vi "Red's Auto Clicker.vi"(8 "error in (no error)":errorcluster) -> (0 "error out":errorcluster)   [LabVIEW 2023]
doc: "Presents an interface to create, edit, save, and execute user-defined macros."
uses:
  CTLs/State Data.ctl
  CTLs/Macro Cluster V3.ctl
  CTLs/Macro Config V3.ctl
  CTLs/Step V3.ctl
  CTLs/Step Type V3.ctl
  CTLs/Hotkey Values.ctl
  CTLs/Refs.ctl
  <vilib>/Utility/miscctls.llb/LVRowAndColumnUnsignedTypeDef.ctl
  CTLs/FGV Actions.ctl
  CTLs/Hotkey Type.ctl
  bd503c13-d10c-440e-ab5e-4e60baef5deb.vi
  <vilib>/Utility/inputDevices.llb/closeKeyboard.vi
  SubVIs/FaKI State Machine/FaKI State Machine.lvlib
panel:
  out "Status":string
  in  "Add Step 2":bool
  in  "Dbl Click":T1
  in  "Macro Steps":i32(listbox)
  out "Abort Hotkey":string caption="Abort Hotkey:"
  out "Metadata":string
  in  "Description":string
  out "Resolutions":cluster{"Width":i16, "Height":i16}[](array[cluster])
  out "n Monitors":i32
  in  "Settings":bool
  in  "Export":bool
  in  "Import":bool
  out "Macro Hotkey":string caption="Macro Hotkey:"
  in  "Delete":bool
  in  "Start/Stop":bool
  in  "N":i32 caption="Times to Repeat\n(-1 = indefinitely)" min=-1
  in  "Activation Type":enum32{"Hotkey", "Automatic"}(radio)
  out "Row":i32
  in  "Clear Steps":bool
  in  "Delete Step":bool
  in  "Insert Step":bool
  in  "Add Step":bool
  in  "Modify Step":bool
  in  "Exit":bool
  in  "Save":bool
  in  "Restore":bool
  in  "Help":bool
  in  "Macro Name":string(combo)
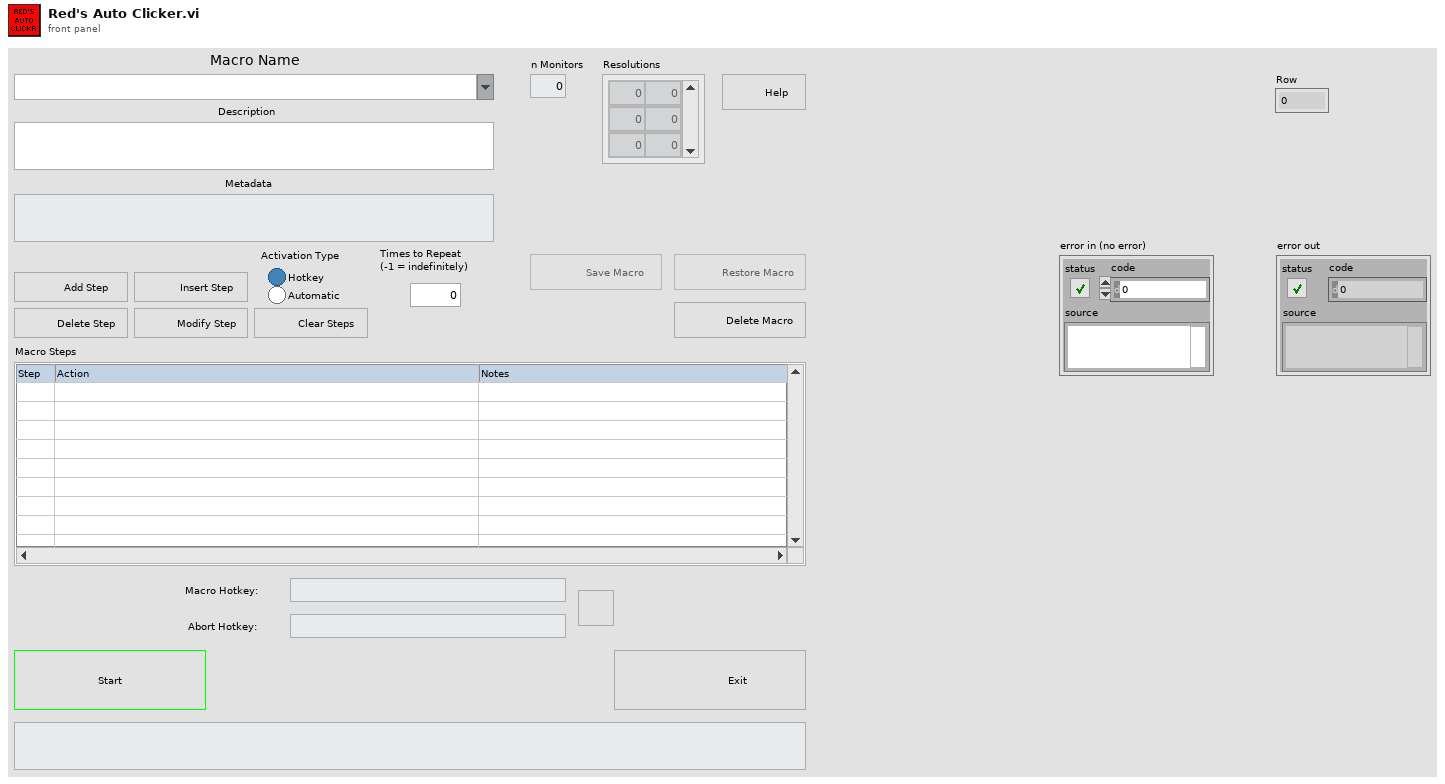
[diagram p1: front panel]
types:
  T1 = cluster{"Insert Before":bool, "Insert After":bool, "Modify Step 2":bool, "Delete Step 2":bool}
  T2 = typedef "LVPoint32TypeDef.ctl" = cluster{"Horizontal":i32, "Vertical":i32}
  T3 = enum32{"Invalid", "Standard", "Closed", "Hidden", "Minimized", "Maximized"}
  T4 = enum32{"invalid app kind", "Development System", "Run Time System", "Student Edition", "Embedded LabVIEW", "Evaluation", "Custom"}
  T5 = typedef "State Data.ctl" = cluster{"Core":cluster{"Current VI Reference":refnum<vi>, "Close Panel on Exit?":bool}, "Macro":cluster{"New":T6, "Saved":T6, "Name":string}, "Step":i32, "n":i32, "Hotkey Values":T10, "Keyboard":refnum<k1>, "Macro Active?":bool, "Macro Names":string[], "Rcount":i32, "Refs":T11, "Resolutions":cluster{"Width":i16, "Height":i16}[], "App Data Dir":path, "Start Time":timestamp}
  T6 = typedef "Macro Cluster V3.ctl" = cluster{"Config":T7, "Steps":T8[]}
  T7 = typedef "Macro Config V3.ctl" = cluster{"Schema Version":string, "Activation Type":enum32{"Hotkey", "Automatic"}, "N":i32, "Description":string, "Resolutions":cluster{"Width":i16, "Height":i16}[], "Date Created":timestamp, "Date Updated":timestamp}
  T8 = typedef "Step V3.ctl" = cluster{"Type":T9, "X":i32, "Y":i32, "Delay":i32, "Key":u8, "Repeat":i32, "RClick?":bool, "App/Window Name":string, "Notes":string}
  T9 = typedef "Step Type V3.ctl" = enum16{"Mouse Move", "Mouse Click", "Key Press", "Wait", "Mouse Down", "Mouse Up", "Key Down", "Key Up", "Run Application", "Maximize Window", "Restore Window", "Minimize Window", "Close Window", "Bring Window to Front", "Send Window to Back"}
  T10 = typedef "Hotkey Values.ctl" = cluster{"Macro Hotkey":enum16{"0", "1", "2", "3", "4", "5", "6", "7", "8", "9", "A", "B", "C", "D", "E", "F", "G", "H", "I", "J", "K", "L", "M", "N", "O", "P", "Q", "R", "S", "T", "U", "V", "W", "X", "Y", "Z", "F1", "F2", "F3", "F4", "F5", "F6", "F7", "F8", "F9", "F10", "F11", "F12", "F13", "F14", "F15", "ADD", "BACK", "BACKSLASH", "CAPITAL", "COMMA", "DECIMAL", "DELETE", "DIVIDE", "DOWN", "END", "EQUALS", "ESCAPE", "GRAVE (`)", "HOME", "INSERT", "LBRACKET", "LCONTROL", "LEFT", "L ALT", "LSHIFT", "LWIN", "MINUS", "MULTIPLY", "NEXT", "NUMLOCK", "NUMPAD_0", "NUMPAD_1", "NUMPAD_2", "NUMPAD_3", "NUMPAD_4", "NUMPAD_5", "NUMPAD_6", "NUMPAD_7", "NUMPAD_8", "NUMPAD_9", "PAUSE", "PERIOD", "PRIOR (PG UP)", "RBRACKET", "RCONTROL", "RETURN", "RIGHT", "R ALT", "RSHIFT", "RWIN", "SCROLL", "SEMICOLON", "SLASH", "SPACE", "SUBTRACT", "TAB", "UP", "ENTER (num pad)", "' (quote)"}[], "Abort Hotkey":enum16{"0", "1", "2", "3", "4", "5", "6", "7", "8", "9", "A", "B", "C", "D", "E", "F", "G", "H", "I", "J", "K", "L", "M", "N", "O", "P", "Q", "R", "S", "T", "U", "V", "W", "X", "Y", "Z", "F1", "F2", "F3", "F4", "F5", "F6", "F7", "F8", "F9", "F10", "F11", "F12", "F13", "F14", "F15", "ADD", "BACK", "BACKSLASH", "CAPITAL", "COMMA", "DECIMAL", "DELETE", "DIVIDE", "DOWN", "END", "EQUALS", "ESCAPE", "GRAVE (`)", "HOME", "INSERT", "LBRACKET", "LCONTROL", "LEFT", "L ALT", "LSHIFT", "LWIN", "MINUS", "MULTIPLY", "NEXT", "NUMLOCK", "NUMPAD_0", "NUMPAD_1", "NUMPAD_2", "NUMPAD_3", "NUMPAD_4", "NUMPAD_5", "NUMPAD_6", "NUMPAD_7", "NUMPAD_8", "NUMPAD_9", "PAUSE", "PERIOD", "PRIOR (PG UP)", "RBRACKET", "RCONTROL", "RETURN", "RIGHT", "R ALT", "RSHIFT", "RWIN", "SCROLL", "SEMICOLON", "SLASH", "SPACE", "SUBTRACT", "TAB", "UP", "ENTER (num pad)", "' (quote)"}[]}
  T11 = typedef "Refs.ctl" = cluster{"Name":refnum<vi>, "Description":refnum<vi>, "Import":refnum<vi>, "Export":refnum<vi>, "Delete":refnum<vi>, "Restore":refnum<vi>, "Save":refnum<vi>, "Start":refnum<vi>, "Steps":refnum<vi>, "Simple Refs":refnum<vi>[]}
  T12 = enum8{"Enabled", "Disabled", "Disabled and Grayed Out"}
  T13 = typedef "LVRowAndColumnUnsignedTypeDef.ctl" = cluster{"Row":u32, "Column":u32}
  T14 = typedef "Hotkey Type.ctl" = enum16{"Macro Hotkey", "Abort Hotkey"}
  T15 = typedef "FGV Actions.ctl" = enum16{"Read", "Write"}
  T16 = cluster{"Current VI Reference":refnum<vi>, "Close Panel on Exit?":bool}
  T17 = enum16{"0", "1", "2", "3", "4", "5", "6", "7", "8", "9", "A", "B", "C", "D", "E", "F", "G", "H", "I", "J", "K", "L", "M", "N", "O", "P", "Q", "R", "S", "T", "U", "V", "W", "X", "Y", "Z", "F1", "F2", "F3", "F4", "F5", "F6", "F7", "F8", "F9", "F10", "F11", "F12", "F13", "F14", "F15", "ADD", "BACK", "BACKSLASH", "CAPITAL", "COMMA", "DECIMAL", "DELETE", "DIVIDE", "DOWN", "END", "EQUALS", "ESCAPE", "GRAVE (`)", "HOME", "INSERT", "LBRACKET", "LCONTROL", "LEFT", "L ALT", "LSHIFT", "LWIN", "MINUS", "MULTIPLY", "NEXT", "NUMLOCK", "NUMPAD_0", "NUMPAD_1", "NUMPAD_2", "NUMPAD_3", "NUMPAD_4", "NUMPAD_5", "NUMPAD_6", "NUMPAD_7", "NUMPAD_8", "NUMPAD_9", "PAUSE", "PERIOD", "PRIOR (PG UP)", "RBRACKET", "RCONTROL", "RETURN", "RIGHT", "R ALT", "RSHIFT", "RWIN", "SCROLL", "SEMICOLON", "SLASH", "SPACE", "SUBTRACT", "TAB", "UP", "ENTER (num pad)", "' (quote)"}[]
  T18 = typedef "LVAllMonitorsDisplayTypeDef.ctl" = cluster{"Bounds":cluster{"Left":i16, "Top":i16, "Right":i16, "Bottom":i16}, "Depth":i16}[]
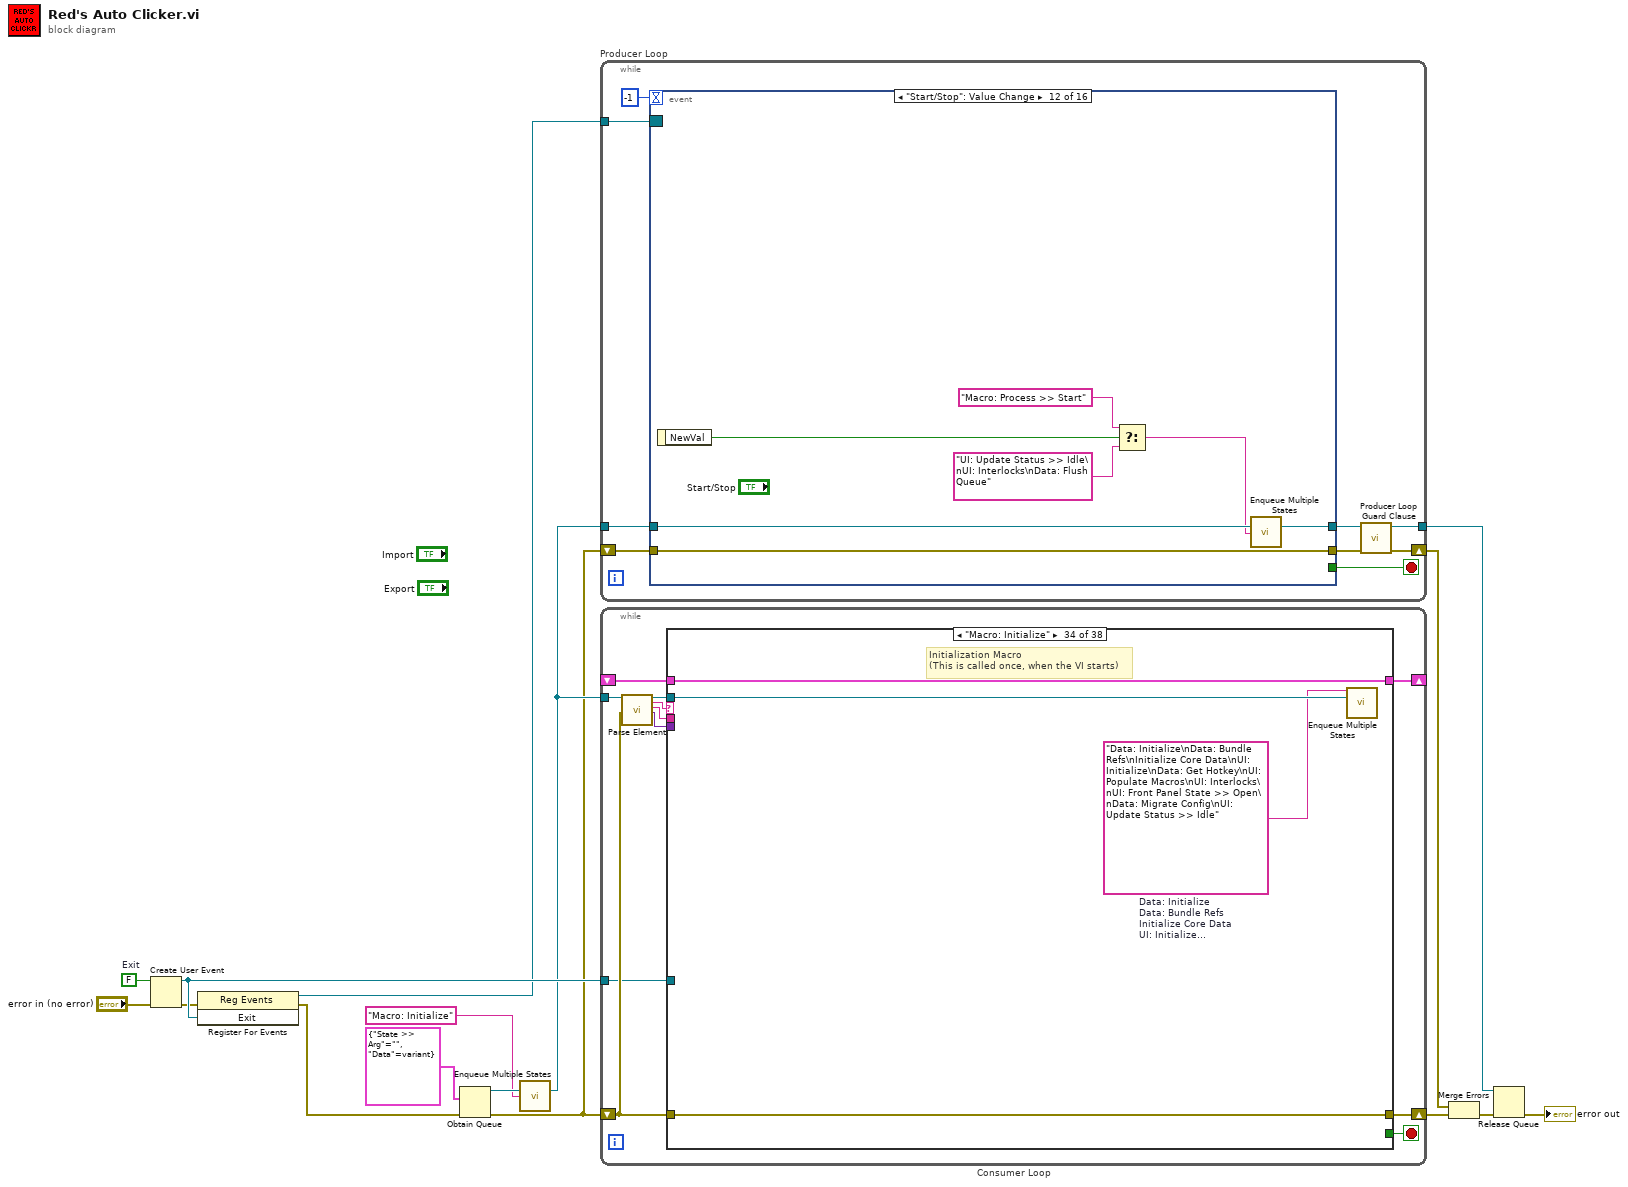
[diagram p0: block diagram]
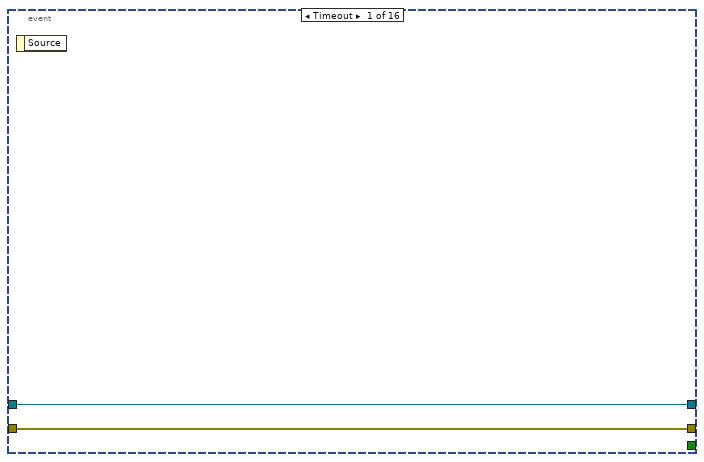
[diagram p2: hidden frame]
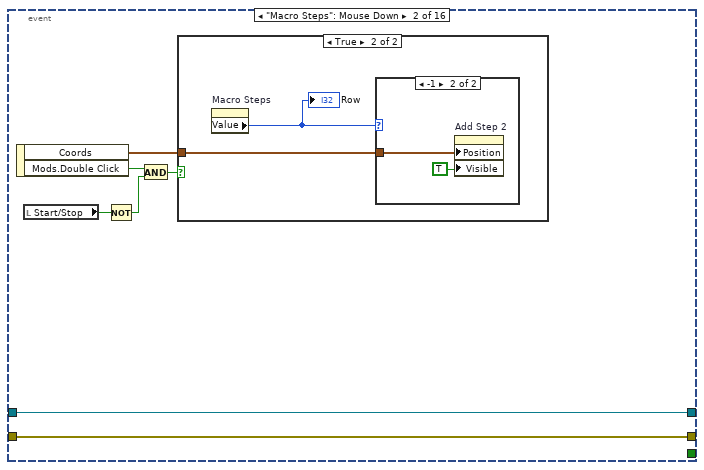
[diagram p3: hidden frame]
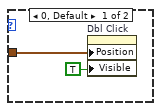
[diagram p5: hidden frame]
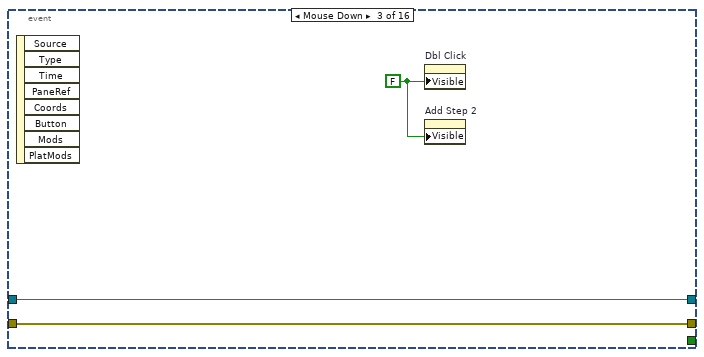
[diagram p6: hidden frame]
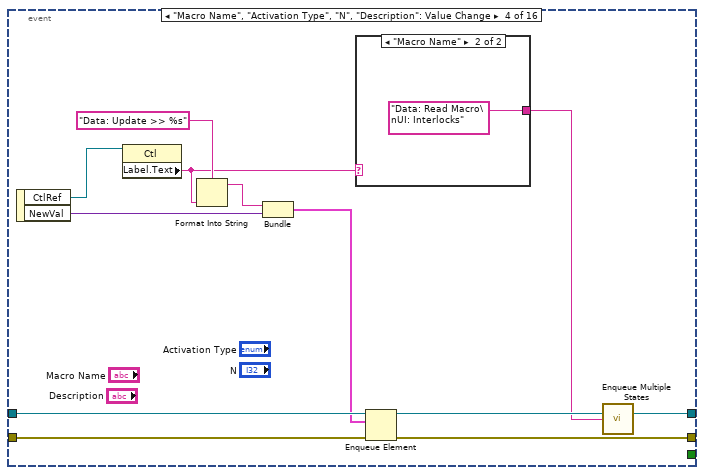
[diagram p7: hidden frame]
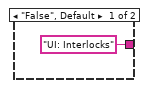
[diagram p8: hidden frame]
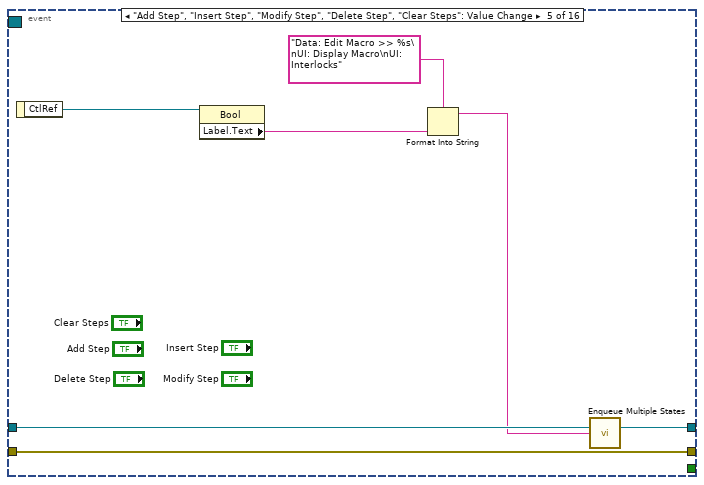
[diagram p9: hidden frame]
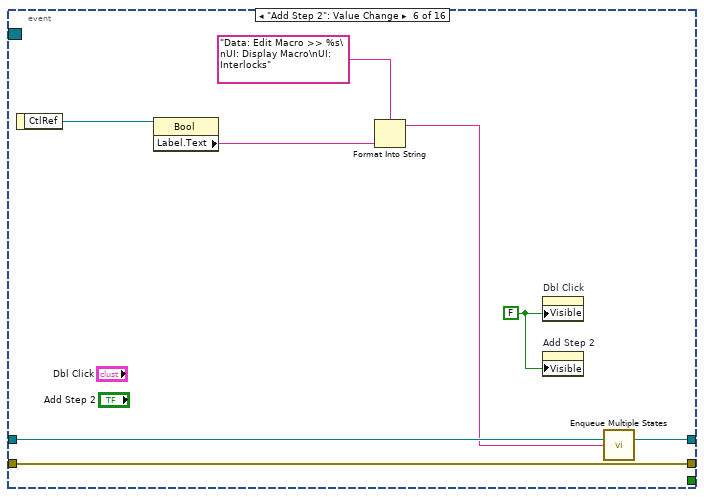
[diagram p10: hidden frame]
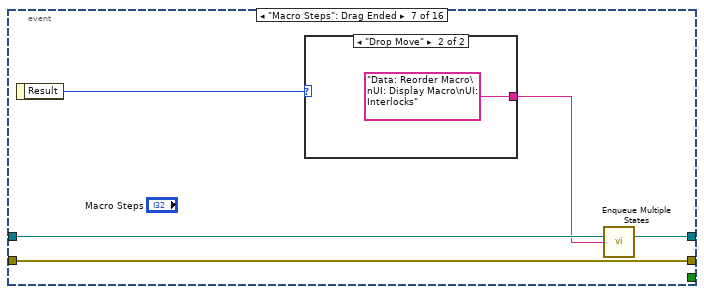
[diagram p11: hidden frame]
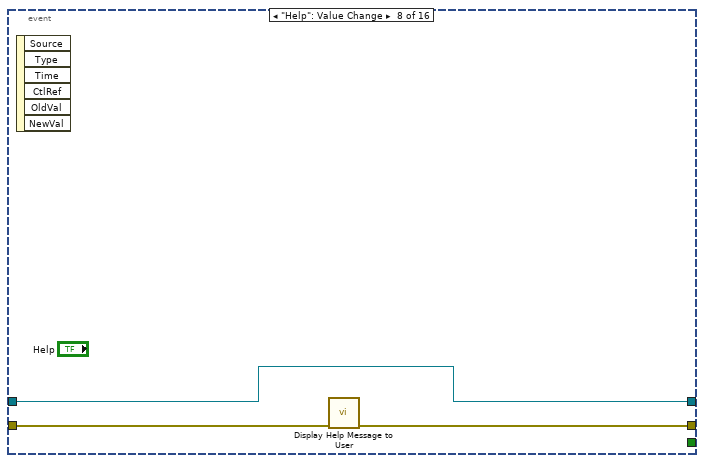
[diagram p13: hidden frame]
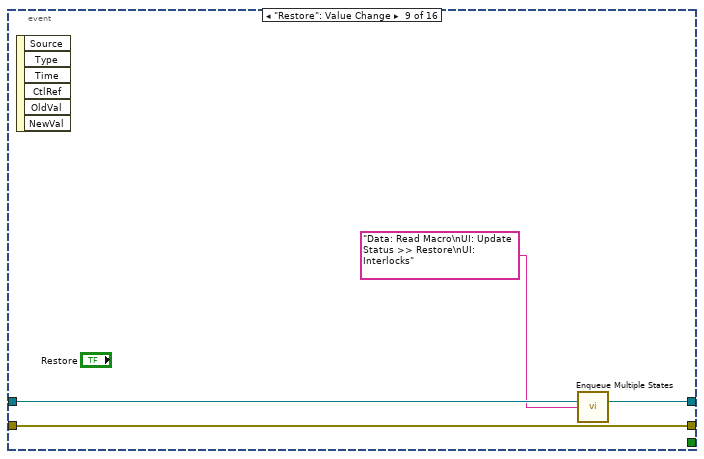
[diagram p14: hidden frame]
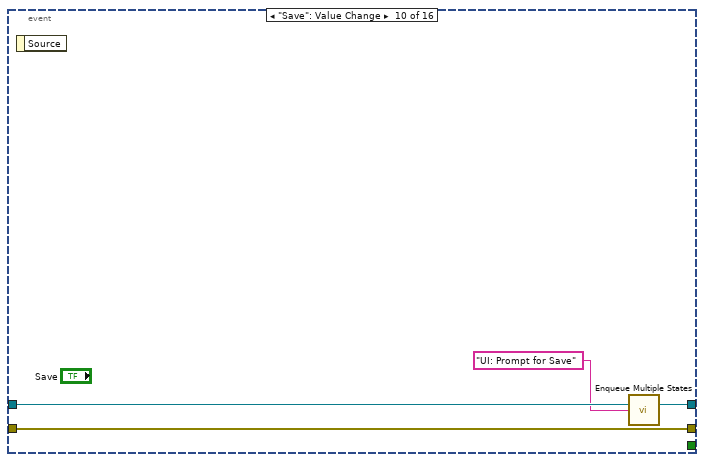
[diagram p15: hidden frame]
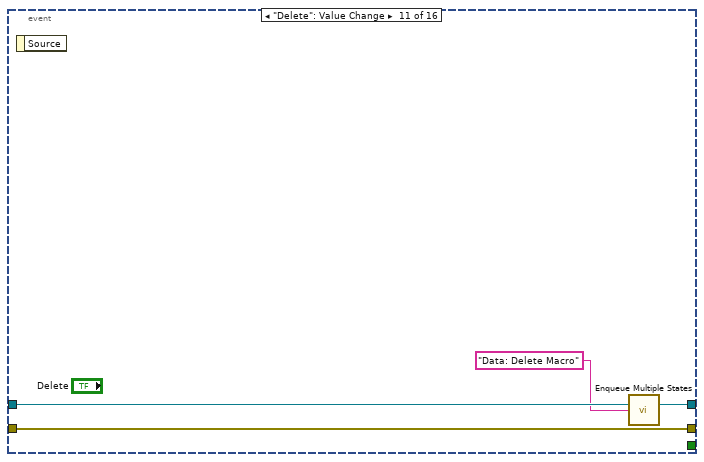
[diagram p16: hidden frame]
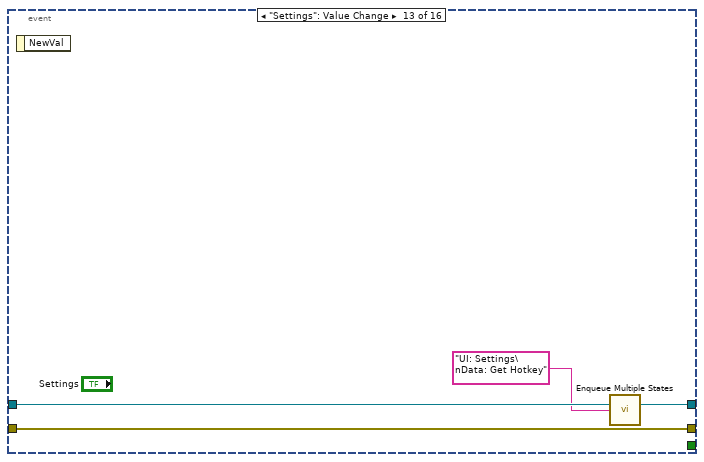
[diagram p17: hidden frame]
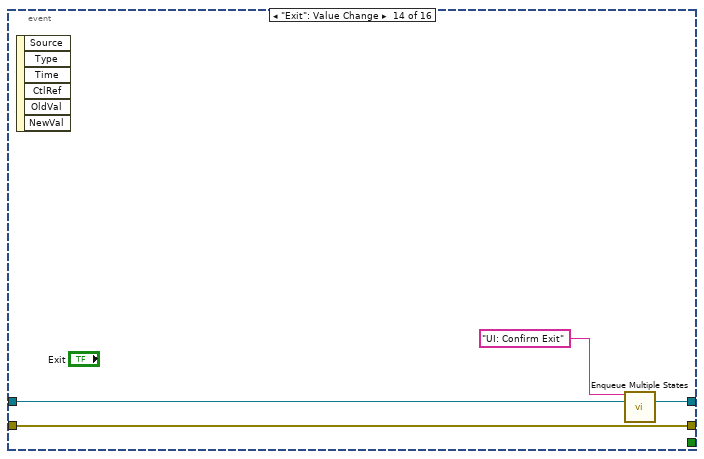
[diagram p18: hidden frame]
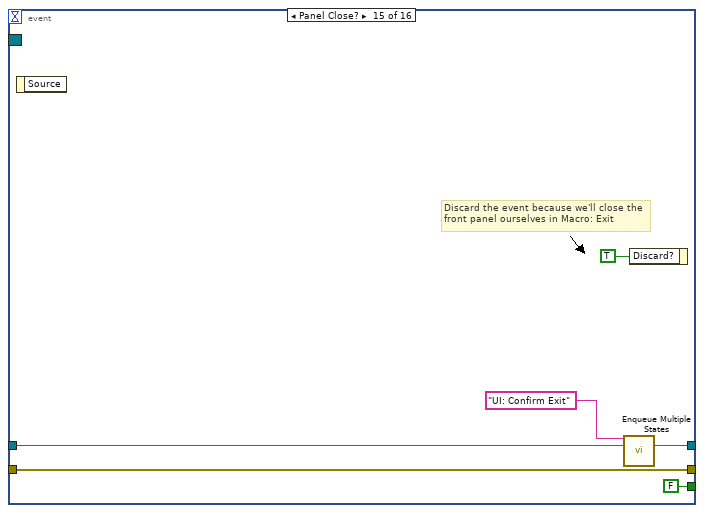
[diagram p19: hidden frame]
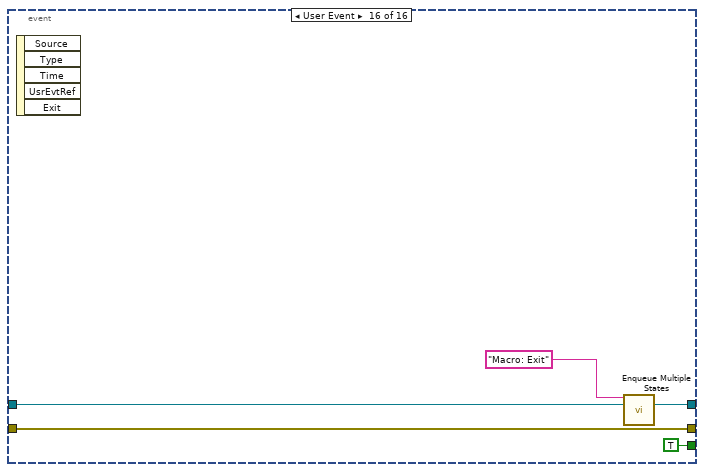
[diagram p20: hidden frame]
diagram:
  w13 = FALSE  # Exit
  n1 = Create User Event(user event datatype=w13, error in="error in (no error)") -> (user event=w16:refnum<user-event>, error out=w12:errorcluster)
  n2 = register-events(error in=w12, w16) -> (reference out=w15:refnum<event-registration>, error out=w14:errorcluster)  [unwired: 1 in]
  n3 = Obtain Queue(element data type=cluster{"State >> Arg":string, "Data":variant} {"State >> Arg"="", "Data"=variant}, error in (no error)=w14) -> (queue out=w6:refnum<queue>, error out=w3:errorcluster)  [unwired: 3 in, 1 out]
  n4 = call "Enqueue Multiple States.vi"("queue in"=w6, "State(s) at Back"="Macro: Initialize") -> ("queue out"=w7:refnum<queue>)  [unwired: 13 in]
  n5 = while "Producer Loop" {
    shift-right: [w25] -> w9
    shift-left: w3 -> [w23]
    tunnel: w15 -> [w19]
    tunnel: w7 -> [w21]
    tunnel: [w24] -> w11
    stop <- w18 stop-if-true
    n6 = event shown="[11] \"Start/Stop\": Value Change" {
      selector: w19 -> [_ _ _ _ _ _ _ _ _ _ _ _ _ _ _ _]
      dyn-events: _ -> [_ _ _ _ _ _ _ _ _ _ _ _ _ _ _ _]
      timeout: -1 ("Timeout") -> [_ _ _ _ _ _ _ _ _ _ _ _ _ _ _ _]
      tunnel: [w27 w34 w43 w51 w64 w72 w77 w80 w85 w89 w93 w100 w104 w108 w114 w119] -> w22
      tunnel: w23 -> [w27 w34 w43 w54 w64 w72 w77 w81 w85 w89 w93 w100 w104 w108 w114 w119]
      tunnel: w21 -> [w26 w32 w42 w48 w62 w69 w76 w79 w83 w88 w92 w96 w102 w106 w111 w117]
      tunnel: [w26 w32 w42 w53 w61 w68 w75 w79 w84 w87 w91 w97 w103 w105 w110 w116] -> w20
      tunnel: [_ _ _ _ _ _ _ _ _ _ _ _ _ _ FALSE TRUE] -> w18
      event Timeout {
        n7 = event-data() -> ()  [unwired: 1 in, 1 out]
      }
      event "Macro Steps": Mouse Down {
        n8 = event-data() -> ("Coords"=w33:T2, "Mods.Double Click"=w29:bool)  [unwired: 1 in]
        n9 = local read "Start/Stop"() -> (w31:bool)
        n10 = Not(x=w31) -> (.not. x?=w30:bool)
        n11 = And(x=w29, y=w30) -> (x .and. y?=w28:bool)
        n12 = case shown="True" w28 {
          tunnel: w33 -> [_ w36]
          frame False {
          }
          frame True {
            n13 = property on="Macro Steps" class="MCListbox (strict)"() -> ("Value"=w35:i32)  [unwired: 2 in, 2 out]
            "Row" <- w35
            n14 = case shown="-1" w35 {
              tunnel: w36 -> [w37 w39]
              frame 0, Default {
                n15 = property on="Dbl Click" class="Clust"("Position"=w37, "Visible"=TRUE) -> ()  [unwired: 2 in, 2 out]
              }
              frame -1 {
                n16 = property on="Add Step 2" class="Bool"("Position"=w39, "Visible"=TRUE) -> ()  [unwired: 2 in, 2 out]
              }
            }
          }
        }
      }
      event Mouse Down {
        w41 = FALSE ("Visible")
        n17 = event-data() -> ()  [unwired: 1 in, 8 out]
        n18 = property on="Dbl Click" class="Clust"("Visible"=w41) -> ()  [unwired: 2 in, 2 out]
        n19 = property on="Add Step 2" class="Bool"("Visible"=w41) -> ()  [unwired: 2 in, 2 out]
      }
      event "Macro Name", "Activation Type", "N", "Description": Value Change {
        n20 = event-data() -> ("CtlRef"=w50:refnum<vi>, "NewVal"=w46:variant)  [unwired: 1 in]
        n21 = property class="Ctl"(reference=w50) -> ("Label.Text"=w45:string)  [unwired: 1 in, 2 out]
        n22 = Format Into String(format string="Data: Update >> %s", w45) -> (resulting string=w47:string)  [unwired: 2 in, 1 out]
        n23 = Bundle(w47, "NewVal"=w46) -> (w44:cluster{string, "NewVal":variant})  [unwired: 1 in]
        n24 = case shown="\"Macro Name\"" w45 {
          tunnel: ["UI: Interlocks" ("string") "Data: Read Macro\nUI: Interlocks" ("string")] -> w52
          frame "False", Default {
          }
          frame "Macro Name" {
          }
        }
        n25 = Enqueue Element(queue=w48, element=w44, error in (no error)=w54) -> (queue out=w55:refnum<queue>, error out=w51:errorcluster)  [unwired: 1 in, 1 out]
        n26 = call "Enqueue Multiple States.vi"("queue in"=w55, "State(s) at Back"=w52) -> ("queue out"=w53:refnum<queue>)  [unwired: 13 in]
      }
      event "Add Step", "Insert Step", "Modify Step", "Delete Step", "Clear Steps": Value Change {
        n27 = event-data() -> ("CtlRef"=w63:refnum<vi>)  [unwired: 1 in]
        n28 = property class="Bool"(reference=w63) -> ("Label.Text"=w60:string)  [unwired: 1 in, 2 out]
        n29 = Format Into String(format string="Data: Edit Macro >> %s\nUI: Display Macro\nUI: Interlocks", w60) -> (resulting string=w58:string)  [unwired: 2 in, 1 out]
        n30 = call "Enqueue Multiple States.vi"("queue in"=w62, "State(s) at Back"=w58) -> ("queue out"=w61:refnum<queue>)  [unwired: 13 in]
      }
      event "Dbl Click.Insert Before", "Dbl Click.Insert After", "Dbl Click.Modify Step 2", "Dbl Click.Delete Step 2", "Add Step 2": Value Change {
        w70 = FALSE ("Visible")
        n31 = event-data() -> ("CtlRef"=w71:refnum<vi>)  [unwired: 1 in]
        n32 = property class="Bool"(reference=w71) -> ("Label.Text"=w66:string)  [unwired: 1 in, 2 out]
        n33 = Format Into String(format string="Data: Edit Macro >> %s\nUI: Display Macro\nUI: Interlocks", w66) -> (resulting string=w65:string)  [unwired: 2 in, 1 out]
        n34 = property on="Dbl Click" class="Clust"("Visible"=w70) -> ()  [unwired: 2 in, 2 out]
        n35 = property on="Add Step 2" class="Bool"("Visible"=w70) -> ()  [unwired: 2 in, 2 out]
        n36 = call "Enqueue Multiple States.vi"("queue in"=w69, "State(s) at Back"=w65) -> ("queue out"=w68:refnum<queue>)  [unwired: 13 in]
      }
      event "Macro Steps": Drag Ended {
        n37 = event-data() -> ("Result"=w73:enum16{"Drop Cancel", "Drop Move", "Drop Copy"})  [unwired: 1 in]
        n38 = case shown="\"Drop Move\"" w73 {
          tunnel: [_ "Data: Reorder Macro\nUI: Display Macro\nUI: Interlocks" ("State(s) at Back")] -> w74
          frame "Drop Cancel", Default {
          }
          frame "Drop Move" {
          }
        }
        n39 = call "Enqueue Multiple States.vi"("queue in"=w76, "State(s) at Back"=w74) -> ("queue out"=w75:refnum<queue>)  [unwired: 13 in]
      }
      event "Help": Value Change {
        n40 = event-data() -> ()  [unwired: 1 in, 6 out]
        n41 = call "Display Help Message to User"("error in (no error)"=w81) -> ("error out"=w80:errorcluster)  [unwired: 9 in, 1 out]
      }
      event "Restore": Value Change {
        n42 = event-data() -> ()  [unwired: 1 in, 6 out]
        n43 = call "Enqueue Multiple States.vi"("queue in"=w83, "State(s) at Back"="Data: Read Macro\nUI: Update Status >> Restore\nUI: Interlocks" ("State(s) at Back (\"\")")) -> ("queue out"=w84:refnum<queue>)  [unwired: 13 in]
      }
      event "Save": Value Change {
        n44 = event-data() -> ()  [unwired: 1 in, 1 out]
        n45 = call "Enqueue Multiple States.vi"("queue in"=w88, "State(s) at Back"="UI: Prompt for Save" ("State(s) at Back (\"\")")) -> ("queue out"=w87:refnum<queue>)  [unwired: 13 in]
      }
      event "Delete": Value Change {
        n46 = event-data() -> ()  [unwired: 1 in, 1 out]
        n47 = call "Enqueue Multiple States.vi"("queue in"=w92, "State(s) at Back"="Data: Delete Macro" ("State(s) at Back (\"\")")) -> ("queue out"=w91:refnum<queue>)  [unwired: 13 in]
      }
      event "Start/Stop": Value Change {
        n48 = event-data() -> ("NewVal"=w99:bool)  [unwired: 1 in]
        n49 = Select(t="Macro: Process >> Start", s=w99, f="UI: Update Status >> Idle\nUI: Interlocks\nData: Flush Queue") -> (s? t:f=w95:string)
        n50 = call "Enqueue Multiple States.vi"("queue in"=w96, "State(s) at Back"=w95) -> ("queue out"=w97:refnum<queue>)  [unwired: 13 in]
      }
      event "Settings": Value Change {
        n51 = event-data() -> ()  [unwired: 1 in, 1 out]
        n52 = call "Enqueue Multiple States.vi"("queue in"=w102, "State(s) at Back"="UI: Settings\nData: Get Hotkey" ("f")) -> ("queue out"=w103:refnum<queue>)  [unwired: 13 in]
      }
      event "Exit": Value Change {
        n53 = event-data() -> ()  [unwired: 1 in, 6 out]
        n54 = call "Enqueue Multiple States.vi"("State(s) at Front"="UI: Confirm Exit", "queue in"=w106) -> ("queue out"=w105:refnum<queue>)  [unwired: 13 in]
      }
      event Panel Close? {
        # "Discard the event because we'll close the front panel ourselves in Macro: Exit"
        n55 = event-data() -> ()  [unwired: 1 in, 1 out]
        n56 = call "Enqueue Multiple States.vi"("State(s) at Front"="UI: Confirm Exit", "queue in"=w111) -> ("queue out"=w110:refnum<queue>)  [unwired: 13 in]
        n57 = event-data("Discard?"=TRUE) -> ()  [unwired: 1 in, 1 out]
      }
      event User Event {
        n58 = event-data() -> ()  [unwired: 1 in, 5 out]
        n59 = call "Enqueue Multiple States.vi"("State(s) at Front"="Macro: Exit", "queue in"=w117) -> ("queue out"=w116:refnum<queue>)  [unwired: 13 in]
      }
    }
    n60 = call "Producer Loop Guard Clause.vi"("error in (no error)"=w22, "queue in"=w20) -> ("error out"=w25:errorcluster, "queue out"=w24:refnum<queue>)  [unwired: 8 in]
  }
  n61 = while "Consumer Loop" {
    shift-right: [w121] -> _
    shift-left: _ -> [w126]
    shift-right: [w128] -> w8
    shift-left: w3 -> [w129]
    tunnel: w7 -> [w130]
    tunnel: w16 -> [w120]
    stop <- w127 stop-if-true
    n62 = call "Parse Element.vi"("queue in"=w130, "error in (no error)"=w129) -> ("queue out"=w125:refnum<queue>, "State"=w124:string, "Arg"=w123:string, "Data"=w122:variant)  [unwired: 14 in]
    n63 = case shown="\"Macro: Initialize\"" w124 {
      selector: w124 -> [_ w133 _ _ _ _ _ _ _ _ _ _ _ _ _ _ _ _ _ _ _ _ _ _ _ _ _ _ _ _ _ _ _ _ _ _ _ _]
      tunnel: w125 -> [_ _ _ _ _ _ _ _ _ _ _ _ _ _ _ w342 w364 w377 _ _ _ _ _ _ _ _ _ w548 w563 _ w586 _ _ w606 w607 w665 _ w683]
      tunnel: w123 -> [_ _ _ w154 _ _ _ _ _ w207 _ w259 _ _ _ _ _ _ _ _ _ w405 w413 _ _ _ w503 _ _ _ _ _ _ _ w611 _ _ _]
      tunnel: w126 -> [w131 w135 w147 w157 w161 w162 _ w185 w197 w208 w257 w260 w310 w315 w330 w338 w361 w378 w386 w387 w391 w408 w415 w485 w490 w501 w504 w547 w566 w574 w585 w595 w601 w604 w608 w670 w672 w676]
      tunnel: [w132 w137 w151 errorcluster {"status"=FALSE, "code"=0, "source"=""} ("error out") w160 w163 w165 w186 w198 w203 w255 w262 w312 w322 w331 w340 w365 w379 w384 w388 w395 w406 w416 w486 w492 w496 w505 w553 w562 w572 w578 w589 w602 w605 w612 w671 w673 w681] -> w128
      tunnel: w129 -> [w132 w136 w151 w156 w160 w163 w171 w186 w196 w206 w249 w262 w312 w322 w332 w341 w366 w379 w383 w388 w395 w407 w417 w486 w493 w496 w505 w550 w567 w573 w578 w593 w602 w605 w612 w671 w673 w682]
      tunnel: [_ _ _ _ TRUE _ _ _ _ _ _ _ _ _ _ _ _ _ _ _ _ _ _ _ _ _ _ _ _ _ _ _ _ _ _ _ _ _] -> w127
      tunnel: w122 -> [_ _ _ w153 _ _ _ _ _ w205 _ _ _ _ _ _ _ _ _ _ _ _ _ _ _ _ _ _ _ _ _ _ _ _ _ _ _ _]
      tunnel: [w131 w135 w152 w157 w161 w162 w166 w184 w197 w204 w256 w261 w311 w321 w327 w339 w361 w378 w386 w387 w389 w408 w415 w485 w491 w501 w504 w547 w566 w574 w585 w595 w601 w604 w610 w670 w672 w675] -> w121
      tunnel: w120 -> [_ _ _ _ _ _ _ _ _ _ _ _ _ _ _ _ _ _ _ _ _ _ _ _ _ _ _ _ _ _ _ w587 _ _ _ _ _ _]
      frame "---------- Core ----------" {
        # "Do not put any code in this frame.\n(it is a separator no-op)"
      }
      frame Default {
        w140 = 42 items=["No error", "Argument error", "Memory is full", "Out of zone", "End of file", "File already open", "Generic file I/O error", "File not found", "File permission error", "Disk is full", "Duplicate path", "Too many files open", "System feature not enabled", "Resource file not found", "Cannot add resource", "Resource not found", "Image not found", "Image memory error", "Pen does not exist", "Config type invalid", "Config token not found", "Config parse error", "Config memory error", "Bad external code format", "Bad external code offset", "External code not present", "Null window", "Destroy window error", "Null menu", "Print aborted", "Bad print record", "Print driver error", "Windows error during printing", "Memory error during printing", "Print dialog error", "Generic print error", "Invalid device refnum", "Device not found", "Device parameter error", "Device unit error", "Cannot open device", "Device call aborted", "Generic error", "Cancelled by user", "Object ID too low", "Object ID too high", "Object not in heap", "Unknown heap", "Unknown object (invalid DefProc)", "Unknown object (DefProc not in table)", "Message out of range", "Invalid (null) method", "Unknown message", "Manager call not supported", "Bad address", "Network operation in progress", "Network operation timed out", "Connection is busy", "Network attribute not supported", "Network error", "Address in use", "System out of memory", "Connection aborted", "Connection refused", "Not connected", "Already connected", "Connection closed", "Initialization error (interapplication manager)", "Bad occurrence", "Wait on unbound occurrence handler", "Occurrence queue overflow", "Datalog type conflict", "Unused", "Unrecognized type (interapplication manager)", "Memory corrupt", "Failed to make temporary DLL", "Old CIN version", "Drag socket not found", "Failed to load drop-object", "Failed to register OLE object", "Failed to release OLE object", "Format specifier type mismatch", "Unknown format specifier", "Too few format specifiers", "Too many format specifiers", "Scan failed", "Newer CIN version", "Error converting to variant", "Runtime menu error", "Password tampered", "Variant attribute not found", "Incompatible variant data type", "Event data is not available", "Event Store is not present", "Occurrence is not found", "Event Queue is not created", "Event info is not available", "Refnum passed is NULL", "Error retrieving Class GUID", "Error retrieving CoClass GUID", "Error retrieving TypeLib GUID.", "Bad built application magic bytes.", "Specific driver is different from the specific driver associated with the Logical Name.", "There is no session opened to the class driver.", "Max Error", "MAX - Error with config objects", "MAX - Error loading configuration", "MAX - Group not supported"]
        # "Current State"
        # "Do not delete, rename, or modify this frame.\n(this is used to capture unhandled states and typos)"
        # "Handle mistyped state name (developer tool)"
        n64 = Format Into String(format string="Software Exception: Unhandled State \"%s\"." ("message"), error in=w136, w133) -> (resulting string=w139:string, error out=w138:errorcluster)  [unwired: 1 in]
        n65 = call <vilib>:"Error Cluster From Error Code.vi"("show call chain? (False)"=TRUE, "error in (no error)"=w138, "error message (\"\")"=w139, "error code (0)"=w140) -> ("error out"=w137:errorcluster)  [unwired: 5 in]
      }
      frame "Initialize Core Data" {
        # "Do not delete, rename, or modify this frame.\n(this is used to determine panel behavior on exit)"
        # "originally closed?"
        # "exe?"
        # "If panel starts closed or is an EXE, then close it when we exit"
        n66 = property class="VI"() -> ("FP.State"=w144:T3)  [unwired: 2 in, 2 out]
        n67 = property class="App"() -> ("App.Kind"=w150:T4)  [unwired: 2 in, 2 out]
        n68 = control-ref of="Current VI Reference"() -> (w145:refnum<vi>)
        n69 = Equal?(x=w144, y=T3."Closed" ("Front Panel Window:State")) -> (x = y?=w142:bool)
        n70 = Equal?(x=w150, y=T4."Run Time System" ("Application:Kind")) -> (x = y?=w148:bool)
        n71 = Or(x=w142, y=w148) -> (x .or. y?=w146:bool)
        n72 = Bundle By Name(cluster=w147, "Core.Current VI Reference"=w145, "Core.Close Panel on Exit?"=w146) -> (w152:T5)
      }
      frame "Error Handler" {
        # "Unhandled Error -- Display it"
        # "Handle any errors here.\nYou can also output any states to clean-up after errors occur"
        # "Clear error"
        n73 = call "Build Error Message.vi"("error in (no error)"=w156, "Data"=w153, "Arg"=w154) -> ("error out"=w155:errorcluster)  [unwired: 8 in]
        n74 = call <vilib>:"General Error Handler.vi"("error in (no error)"=w155) -> ()  [unwired: 10 in, 5 out]
      }
      frame "Exit" {
        # "Do not put any code in this frame.\n(No errors that occur here will be handled.)"
      }
      frame "---------- Data ----------" {
        # "Do not put any code in this frame.\n(It is a separator no-op. You can make a copy of this frame to create a new Data frame)"
      }
      frame "Data: Initialize" {
        w167 = T16 {"Current VI Reference"=refnum, "Close Panel on Exit?"=FALSE}  # Core
        # "Initialize the shift-register data, here."
        n75 = call <vilib>:"Intialize Keyboard.vi"("error in (no error)"=w171) -> ("error out"=w170:errorcluster, "device ID"=w168:refnum<k1>)  [unwired: 9 in]
        n76 = call "App Data Directory.vi"("error in (no error)"=w170) -> ("error out"=w165:errorcluster, "App Data Directory"=w164:path)  [unwired: 9 in]
        n77 = Bundle By Name(cluster=T5 {"Core"={"Current VI Reference"=refnum, "Close Panel on Exit?"=FALSE}, "Macro"={"New"={"Config"={"Schema Version"="", "Activation Type"=enum."Hotkey", "N"=0, "Description"="", "Resolutions"=[], "Date Created"=timestamp(0 s since 1904-01-01), "Date Updated"=timestamp(0 s since 1904-01-01)}, "Steps"=[]}, "Saved"={"Config"={"Schema Version"="", "Activation Type"=enum."Hotkey", "N"=0, "Description"="", "Resolutions"=[], "Date Created"=timestamp(0 s since 1904-01-01), "Date Updated"=timestamp(0 s since 1904-01-01)}, "Steps"=[]}, "Name"=""}, "Step"=0, "n"=0, "Hotkey Values"={"Macro Hotkey"=[], "Abort Hotkey"=[]}, "Keyboard"=refnum, "Macro Active?"=FALSE, "Macro Names"=[], "Rcount"=0, "Refs"={"Name"=refnum, "Description"=refnum, "Import"=refnum, "Export"=refnum, "Delete"=refnum, "Restore"=refnum, "Save"=refnum, "Start"=refnum, "Steps"=refnum, "Simple Refs"=[]}, "Resolutions"=[], "App Data Dir"=path "", "Start Time"=timestamp(0 s since 1904-01-01)}, "Core"=w167, "Keyboard"=w168, "App Data Dir"=w164) -> (w166:T5)
      }
      frame "Data: Bundle Refs" {
        n78 = control-ref of="Activation Type"() -> (w189:refnum<vi>)
        n79 = control-ref of="Macro Name"() -> (w187:refnum<vi>)
        n80 = control-ref of="Add Step"() -> (w194:refnum<vi>)
        n81 = control-ref of="Delete Step"() -> (w192:refnum<vi>)
        n82 = control-ref of="Insert Step"() -> (w191:refnum<vi>)
        n83 = control-ref of="Modify Step"() -> (w193:refnum<vi>)
        n84 = control-ref of="Clear Steps"() -> (w190:refnum<vi>)
        n85 = control-ref of="Settings"() -> (w175:refnum<vi>)
        n86 = control-ref of="Help"() -> (w173:refnum<vi>)
        n87 = control-ref of="N"() -> (w188:refnum<vi>)
        n88 = control-ref of="Macro Steps"() -> (w172:refnum<vi>)
        n89 = control-ref of="Macro Name"() -> (w183:refnum<vi>)
        n90 = control-ref of="Import"() -> (w181:refnum<vi>)
        n91 = control-ref of="Export"() -> (w180:refnum<vi>)
        n92 = control-ref of="Delete"() -> (w179:refnum<vi>)
        n93 = control-ref of="Restore"() -> (w178:refnum<vi>)
        n94 = control-ref of="Save"() -> (w177:refnum<vi>)
        n95 = control-ref of="Start/Stop"() -> (w176:refnum<vi>)
        n96 = control-ref of="Description"() -> (w182:refnum<vi>)
        n97 = Build Array(w194, w192, w191, w193, w190, w189, w188, w187, w175, w173) -> (w174:refnum<vi>[])
        n98 = Bundle By Name(cluster=w185, "Refs.Name"=w183, "Refs.Description"=w182, "Refs.Import"=w181, "Refs.Export"=w180, "Refs.Delete"=w179, "Refs.Restore"=w178, "Refs.Save"=w177, "Refs.Start"=w176, "Refs.Steps"=w172, "Refs.Simple Refs"=w174) -> (w184:T5)
      }
      frame "Data: Migrate Config" {
        n99 = Unbundle By Name(w197) -> ("App Data Dir"=w195:path)
        n100 = call "Config Paths.vi"("error in (no error)"=w196) -> ("error out"=w202:errorcluster, "Process Config"=w201:path, "Global Config"=w199:path)  [unwired: 8 in]
        n101 = call "Migrate Process Config.vi"("error in (no error)"=w202, "Old Process Config"=w201, "App Data Directory"=w195) -> ("error out"=w200:errorcluster)  [unwired: 8 in]
        n102 = call "Migrate Global Config.vi"("error in (no error)"=w200, "Old Global Config"=w199, "App Data Directory"=w195) -> ("error out"=w198:errorcluster)  [unwired: 8 in]
      }
      frame "Data: Update" {
        n103 = case shown="\"Macro Name\"" w207 {
          tunnel: w208 -> [w209 w214 w222 w229 w236 w243]
          tunnel: w206 -> [w210 w218 w225 w232 w239 w246]
          tunnel: w205 -> [_ w217 w224 w231 w238 w245]
          tunnel: [w209 w213 w221 w228 w235 w242] -> w204
          tunnel: [w210 w212 w220 w227 w234 w241] -> w203
          frame "False", Default {
          }
          frame "Macro Name" {
            n104 = Variant To Data(error in=w218, type="", Variant=w217) -> (data=w215:string, error out=w212:errorcluster)
            n105 = property on="Restore" class="Bool"("DisabledEnum"=T12."Disabled and Grayed Out" ("Disabled")) -> ()  [unwired: 2 in, 2 out]
            n106 = Bundle By Name(cluster=w214, "Macro.Name"=w215) -> (w213:T5)
          }
          frame "Activation Type" {
            n107 = Variant To Data(error in=w225, type=enum32{"Hotkey", "Automatic"}."Hotkey" ("FP CTLs.Type"), Variant=w224) -> (data=w223:enum32{"Hotkey", "Automatic"}, error out=w220:errorcluster)
            n108 = Bundle By Name(cluster=w222, "Macro.New.Config.Activation Type"=w223) -> (w221:T5)
          }
          frame "N" {
            n109 = Variant To Data(error in=w232, type=0 ("FP CTLs.N"), Variant=w231) -> (data=w230:i32, error out=w227:errorcluster)
            n110 = Bundle By Name(cluster=w229, "Macro.New.Config.N"=w230) -> (w228:T5)
          }
          frame "Description" {
            n111 = Variant To Data(error in=w239, type="" ("FP CTLs.N"), Variant=w238) -> (data=w237:string, error out=w234:errorcluster)
            n112 = Bundle By Name(cluster=w236, "Macro.New.Config.Description"=w237) -> (w235:T5)
          }
          frame "Macro Active?" {
            n113 = Variant To Data(error in=w246, type=FALSE, Variant=w245) -> (data=w244:bool, error out=w241:errorcluster)
            n114 = Bundle By Name(cluster=w243, "Macro Active?"=w244) -> (w242:T5)
          }
        }
      }
      frame "Data: Get Hotkey" {
        n115 = call "App Config INI.vi"("error in (no error)"=w249) -> ("error out"=w248:errorcluster, "App Config"=w247:path)  [unwired: 9 in]
        n116 = call "Get Hotkey.vi"("error in (no error)"=w248, "File Path"=w247) -> ("error out"=w255:errorcluster, "Hotkey Values"=w253:T10)  [unwired: 8 in]
        n117 = Unbundle By Name(w253) -> ("Macro Hotkey"=w252:T17, "Abort Hotkey"=w250:T17)
        n118 = Bundle By Name(cluster=w257, "Hotkey Values"=w253) -> (w256:T5)
        n119 = call "Convert Hotkey to String.vi"("Hotkey"=w252) -> ("String"=→"Macro Hotkey":string)  [unwired: 10 in]
        n120 = call "Convert Hotkey to String.vi"("Hotkey"=w250) -> ("String"=→"Abort Hotkey":string)  [unwired: 10 in]
      }
      frame "Data: Edit Macro" {
        n121 = local read "Row"() -> (w258:i32)
        n122 = in-place {
          in-place-border: w259 -> [w264]
          in-place-border: w258 -> [w263]
          n123 = in-place-cluster #1(w260) -> ("Macro.New.Steps"=w266:T8[])
          n124 = case shown="\"Add Step\"" w264 {
            tunnel: w266 -> [w267 w270 w273 w276 w279 w282 w286 w291 w295 w299 w301]
            tunnel: [w267 w269 w272 w275 w278 w281 w285 w290 w294 w298 w300] -> w265
            tunnel: w263 -> [_ _ _ _ _ _ w283 w288 w292 w296 _]
            frame Default {
            }
            frame "Add Step" {
              n125 = call "Alter Macro.vi"("Action"=enum16{"Add", "Insert", "Modify", "Delete"}."Add", "Steps in"=w270) -> ("Steps out"=w269:T8[])  [unwired: 9 in]
            }
            frame "Insert Step" {
              n126 = call "Alter Macro.vi"("Action"=enum16{"Add", "Insert", "Modify", "Delete"}."Insert", "Steps in"=w273) -> ("Steps out"=w272:T8[])  [unwired: 9 in]
            }
            frame "Modify Step" {
              n127 = call "Alter Macro.vi"("Action"=enum16{"Add", "Insert", "Modify", "Delete"}."Modify", "Steps in"=w276) -> ("Steps out"=w275:T8[])  [unwired: 9 in]
            }
            frame "Delete Step" {
              n128 = call "Alter Macro.vi"("Action"=enum16{"Add", "Insert", "Modify", "Delete"}."Delete", "Steps in"=w279) -> ("Steps out"=w278:T8[])  [unwired: 9 in]
            }
            frame "Add Step 2" {
              n129 = call "Alter Macro V2.vi"("Action"=enum16{"Add", "Insert", "Modify", "Delete"}."Add", "Steps in"=w282) -> ("Steps out"=w281:T8[])  [unwired: 9 in]
            }
            frame "Insert Before" {
              n130 = call "Alter Macro V2.vi"("Action"=enum16{"Add", "Insert", "Modify", "Delete"}."Insert", "Step"=w283, "Steps in"=w286) -> ("Steps out"=w285:T8[])  [unwired: 8 in]
            }
            frame "Insert After" {
              n131 = Increment(x=w288) -> (x+1=w287:i32)
              n132 = call "Alter Macro V2.vi"("Action"=enum16{"Add", "Insert", "Modify", "Delete"}."Insert", "Step"=w287, "Steps in"=w291) -> ("Steps out"=w290:T8[])  [unwired: 8 in]
            }
            frame "Modify Step 2" {
              n133 = call "Alter Macro V2.vi"("Action"=enum16{"Add", "Insert", "Modify", "Delete"}."Modify", "Step"=w292, "Steps in"=w295) -> ("Steps out"=w294:T8[])  [unwired: 8 in]
            }
            frame "Delete Step 2" {
              n134 = call "Alter Macro V2.vi"("Action"=enum16{"Add", "Insert", "Modify", "Delete"}."Delete", "Step"=w296, "Steps in"=w299) -> ("Steps out"=w298:T8[])  [unwired: 8 in]
            }
            frame "Clear Steps" {
              n135 = call "Confirm Clear"() -> ("OK"=w302:bool)  [unwired: 10 in, 1 out]
              n136 = case shown="False" w302 {
                tunnel: w301 -> [w303 _]
                tunnel: [w303 _] -> w300
                frame False {
                }
                frame True {
                  n137 = property on="Macro Steps" class="MCListbox (strict)"("TopLeft"=T13 {"Row"=0, "Column"=0} ("Index Values")) -> ()  [unwired: 2 in, 2 out]
                }
              }
            }
          }
          n138 = in-place-cluster #1("Macro.New.Steps"=w265) -> (w261:T5)
        }
      }
      frame "Data: Bundle Macro" {
        n139 = Unbundle By Name(w310) -> ("Resolutions"=w309:cluster{"Width":i16, "Height":i16}[], "Macro.New.Config.Date Created"=w307:timestamp)
        n140 = Get Date/Time In Seconds() -> (seconds since 1Jan1904=w305:timestamp)
        n141 = Not Equal To 0?(x=w307) -> (x != 0?=w308:bool)
        n142 = Select(t=w307, s=w308, f=w305) -> (s? t:f=w306:timestamp)
        n143 = Bundle By Name(cluster=w310, "Macro.New.Config.Resolutions"=w309, "Macro.New.Config.Date Created"=w306, "Macro.New.Config.Date Updated"=w305) -> (w311:T5)
      }
      frame "Data: Reorder Macro" {
        n144 = property on="Macro Steps" class="MCListbox (strict)"() -> ("ItemNames"=w320:string[][])  [unwired: 2 in, 2 out]
        n145 = Index Array(array=w320, index (col)=0 ("disabled index (col)")) -> (element=w318:string[])  [unwired: 1 in]
        n146 = Unbundle By Name(w315) -> ("Macro.New.Steps"=w314:T8[])
        n147 = Decimal String To Number(string=w318) -> (number=w317:i32[])  [unwired: 2 in, 1 out]
        n148 = Decrement(x=w317) -> (x-1=w316:i32[])
        n149 = for {
          tunnel: w316 -> [w323] mode=indexing
          tunnel: w314 -> [w325]
          tunnel: [w324] -> w313 mode=indexing
          n150 = Index Array(array=w325, index=w323) -> (element=w324:T8)
        }
        n151 = Bundle By Name(cluster=w315, "Macro.New.Steps"=w313) -> (w321:T5)
      }
      frame "Data: Save Macro" {
        n152 = Unbundle By Name(w330) -> ("Macro.New"=w326:T6, "Macro.Name"=w329:string, "App Data Dir"=w328:path)
        n153 = call "Save Macro.vi"("Macro Name"=w329, "error in (no error)"=w332, "Macro Cluster"=w326, "App Data Directory"=w328) -> ("error out"=w331:errorcluster)  [unwired: 7 in]
        n154 = Bundle By Name(cluster=w330, "Macro.Saved"=w326) -> (w327:T5)
      }
      frame "Data: Read Macro" {
        n155 = Unbundle By Name(w338) -> ("Macro Names"=w337:string[], "Macro.Name"=w336:string, "App Data Dir"=w333:path)
        n156 = Search 1D Array(1D array=w337, element=w336) -> (index of element=w335:i32)  [unwired: 1 in]
        n157 = in-place {
          in-place-border: w341 -> [w351]
          in-place-border: [w350] -> w340
          in-place-border: w336 -> [w349]
          in-place-border: w335 -> [w348]
          in-place-border: w333 -> [w344]
          n158 = in-place-cluster #2(w338) -> ("Macro.New"=w347:T6)  [unwired: 1 out]
          n159 = case shown="0, Default" w348 {
            tunnel: w351 -> [w356 w359]
            tunnel: [w355 w359] -> w350
            tunnel: w349 -> [w354 _]
            tunnel: w347 -> [_ w358]
            tunnel: [w353 _] -> w346
            tunnel: [w353 w357] -> w345
            tunnel: w344 -> [w352 _]
            frame 0, Default {
              n160 = call "Read Macro.vi"("error in (no error)"=w356, "Macro Name"=w354, "App Data Directory"=w352) -> ("error out"=w355:errorcluster, "Macro"=w353:T6)  [unwired: 7 in]
            }
            frame -1 {
              n161 = call "Clear Macro Data.vi"("Macro"=w358) -> ("Macro out"=w357:T6)  [unwired: 10 in]
            }
          }
          n162 = in-place-cluster #2("Macro.New"=w345, "Macro.Saved"=w346) -> (w339:T5)
        }
        n163 = property on="Macro Steps" class="MCListbox (strict)"("TopLeft"=T13 {"Row"=0, "Column"=0} ("Index Values")) -> ()  [unwired: 2 in, 2 out]
        n164 = call "Enqueue Multiple States.vi"("queue in"=w342, "State(s) at Back"="UI: Display Macro" ("State(s) at Back (\"\")")) -> ()  [unwired: 13 in, 1 out]
      }
      frame "Data: Delete Macro" {
        n165 = Unbundle By Name(w361) -> ("Macro.Name"=w362:string, "App Data Dir"=w360:path)
        n166 = call "Perm Delete?"("error in (no error)"=w366) -> ("error out"=w367:errorcluster, "Delete"=w368:bool)  [unwired: 9 in]
        n167 = case shown="True" w368 {
          tunnel: w367 -> [w369 w371]
          tunnel: [w369 w375] -> w365
          tunnel: [_ "UI: Update Status >> Delete\nUI: Populate Macros" ("State(s) at Back (\"\")")] -> w363
          tunnel: w362 -> [_ w373]
          tunnel: w360 -> [_ w372]
          frame False {
          }
          frame True {
            n168 = call "Delete Macro.vi"("Macro Name"=w373, "error in (no error)"=w371, "App Data Directory"=w372) -> ("error out"=w376:errorcluster)  [unwired: 8 in]
            n169 = property on="Macro Name" class="CmbBox"(error in=w376, "Val(Sgnl)"="") -> (error out=w375:errorcluster)  [unwired: 1 in, 1 out]
          }
        }
        n170 = call "Enqueue Multiple States.vi"("queue in"=w364, "State(s) at Back"=w363) -> ()  [unwired: 13 in, 1 out]
      }
      frame "Data: Flush Queue" {
        n171 = Flush Queue(queue=w377) -> ()  [unwired: 1 in, 3 out]
      }
      frame "Data: Cleanup" {
        # "Cleanup any data and references, here.\n(this is called automatically, by the Macro: Exit)"
        n172 = Unbundle By Name(w386) -> ("Core.Current VI Reference"=w385:refnum<vi>, "Keyboard"=w380:refnum<k1>)
        n173 = Close Reference(reference=w385, error in (no error)=w383) -> (error out=w381:errorcluster)
        n174 = call-poly <vilib>:"Close Input Device.vi"("error in (no error)"=w381, "device ID"=w380) -> ("error out"=w382:errorcluster)  [unwired: 8 in]
        n175 = invoke class="VI" method="Default Vals.Reinit All"(error in=w382) -> (error out=w384:errorcluster)  [unwired: 2 in, 2 out]
      }
      frame "---------- UI ----------" {
        # "Do not put any code in this frame.\n(It is a separator no-op. You can make a copy of this frame to create a new UI frame)"
      }
      frame "UI: Initialize" {
        w396 = T12."Disabled and Grayed Out" ("Disabled")
        # "Initialize the User Interface, here.\n(this is called automatically, by the Macro: Init)"
        n176 = property class="App"() -> ("Disp.AllMonitors"=w392:T18)  [unwired: 2 in, 2 out]
        n177 = for {
          tunnel: w392 -> [w404] mode=indexing
          tunnel: [w403] -> w390 mode=indexing
          n178 = Unbundle By Name(w404) -> ("Bounds.Right"=w402:i16, "Bounds.Left"=w400:i16, "Bounds.Bottom"=w401:i16, "Bounds.Top"=w399:i16)
          n179 = Subtract(x=w402, y=w400) -> (x-y=w397:i16)
          n180 = Subtract(x=w401, y=w399) -> (x-y=w398:i16)
          n181 = Bundle(w397, w398) -> (w403:cluster{i16, i16})  [unwired: 1 in]
        }
        "Resolutions" <- w390
        n182 = Array Size(array=w392) -> (size(s)=→"n Monitors":i32)
        n183 = property on="Start/Stop" class="Bool (strict)"("DisabledEnum"=w396) -> ()  [unwired: 2 in, 2 out]
        n184 = property on="Restore" class="Bool"("DisabledEnum"=w396) -> ()  [unwired: 2 in, 2 out]
        n185 = property on="Save" class="Bool"("DisabledEnum"=w396) -> ()  [unwired: 2 in, 2 out]
        n186 = property on="Start/Stop" class="Bool (strict)"("Colors [4]"=cluster{u32, u32}[] [{65280, 65280}, {16711680, 16711680}, {4424887, 6618880}, {4424887, 16711680}, {4424887, 12648384}, {4424887, 16761024}]) -> ()  [unwired: 2 in, 2 out]
        n187 = Bundle By Name(cluster=w391, "Resolutions"=w390) -> (w389:T5)
      }
      frame "UI: Cursor Set" {
        # "Argument"
        # "Set and Unset Cursor Busy.\n(Usage: \"UI: Cursor Set >> Busy|Idle\")"
        n188 = case shown="\"Idle\", Default" w405 {
          tunnel: w407 -> [w410 w412]
          tunnel: [w409 w411] -> w406
          frame "Idle", Default {
            n189 = call <vilib>:"Unset Busy.vi"("error in (no error)"=w410) -> ("error out"=w409:errorcluster)  [unwired: 10 in]
          }
          frame "Busy" {
            n190 = call <vilib>:"Set Busy.vi"("error in (no error)"=w412) -> ("error out"=w411:errorcluster)  [unwired: 9 in, 1 out]
          }
        }
      }
      frame "UI: Front Panel State" {
        # "Argument"
        # "Set Front Panel Open or Closed\n(Usage: \"UI: Front Panel State >> Open|Close\")"
        n191 = Unbundle By Name(w415) -> ("Core.Current VI Reference"=w414:refnum<vi>)
        n192 = case shown="\"Open\", \"Standard\", Default" w413 {
          tunnel: w417 -> [w423 w438 w449 w462 w475]
          tunnel: [w425 w439 w451 w464 w477] -> w416
          tunnel: w414 -> [w424 w436 w450 w463 w476]
          frame "Open", "Standard", Default {
            w418 = T3."Standard" ("State")
            n193 = property class="VI"(reference=w424, error in=w423) -> (reference out=w421:refnum<vi>, error out=w422:errorcluster, "FP.State"=w420:T3)
            n194 = Not Equal?(x=w420, y=w418) -> (x != y?=w419:bool)
            n195 = case shown="True" w419 {
              tunnel: [w429 w431] -> w425
              tunnel: w422 -> [w428 w431]
              tunnel: w421 -> [w427 _]
              tunnel: w418 -> [w426 _]
              frame True {
                n196 = invoke class="VI" method="FP.Open"(reference=w427, error in=w428, "Activate"=TRUE, "State"=w426) -> (error out=w429:errorcluster)  [unwired: 1 in, 4 out]
              }
              frame False {
              }
            }
          }
          frame "Close", "Closed" {
            n197 = property class="VI"(reference=w436, error in=w438) -> (reference out=w435:refnum<vi>, error out=w437:errorcluster, "FP.State"=w433:T3)
            n198 = Not Equal?(x=w433, y=T3."Closed" ("Front Panel Window:State")) -> (x != y?=w432:bool)
            n199 = case shown="True" w432 {
              tunnel: [w440 w443] -> w439
              tunnel: w437 -> [w440 w442]
              tunnel: w435 -> [_ w441]
              frame False {
              }
              frame True {
                n200 = invoke class="VI" method="FP.Close"(reference=w441, error in=w442) -> (error out=w443:errorcluster)  [unwired: 1 in, 2 out]
              }
            }
          }
          frame "Hidden", "Hide" {
            w444 = T3."Hidden" ("State")
            n201 = property class="VI"(reference=w450, error in=w449) -> (reference out=w447:refnum<vi>, error out=w448:errorcluster, "FP.State"=w446:T3)
            n202 = Not Equal?(x=w446, y=w444) -> (x != y?=w445:bool)
            n203 = case shown="True" w445 {
              tunnel: [w455 w456] -> w451
              tunnel: w448 -> [w454 w456]
              tunnel: w447 -> [w453 _]
              tunnel: w444 -> [w452 _]
              frame True {
                n204 = invoke class="VI" method="FP.Open"(reference=w453, error in=w454, "State"=w452) -> (error out=w455:errorcluster)  [unwired: 2 in, 4 out]
              }
              frame False {
              }
            }
          }
          frame "Minimize", "Minimized" {
            w457 = T3."Minimized" ("State")
            n205 = property class="VI"(reference=w463, error in=w462) -> (reference out=w460:refnum<vi>, error out=w461:errorcluster, "FP.State"=w459:T3)
            n206 = Not Equal?(x=w459, y=w457) -> (x != y?=w458:bool)
            n207 = case shown="True" w458 {
              tunnel: [w468 w469] -> w464
              tunnel: w461 -> [w467 w469]
              tunnel: w460 -> [w466 _]
              tunnel: w457 -> [w465 _]
              frame True {
                n208 = invoke class="VI" method="FP.Open"(reference=w466, error in=w467, "State"=w465) -> (error out=w468:errorcluster)  [unwired: 2 in, 4 out]
              }
              frame False {
              }
            }
          }
          frame "Maximize", "Maximized" {
            w470 = T3."Maximized" ("State")
            n209 = property class="VI"(reference=w476, error in=w475) -> (reference out=w473:refnum<vi>, error out=w474:errorcluster, "FP.State"=w472:T3)
            n210 = Not Equal?(x=w472, y=w470) -> (x != y?=w471:bool)
            n211 = case shown="True" w471 {
              tunnel: [w481 w482] -> w477
              tunnel: w474 -> [w480 w482]
              tunnel: w473 -> [w479 _]
              tunnel: w470 -> [w478 _]
              frame True {
                n212 = invoke class="VI" method="FP.Open"(reference=w479, error in=w480, "State"=w478) -> (error out=w481:errorcluster)  [unwired: 2 in, 4 out]
              }
              frame False {
              }
            }
          }
        }
      }
      frame "UI: Interlocks" {
        n213 = Unbundle By Name(w485) -> ("Refs"=w484:T11, "Macro"=w483:cluster{"New":T6, "Saved":T6, "Name":string})
        n214 = call "UI Interlocks.vi"("Macro"=w483, "Refs"=w484) -> ()  [unwired: 10 in]
      }
      frame "UI: Populate Macros" {
        n215 = Unbundle By Name(w490) -> ("App Data Dir"=w488:path)
        n216 = call "Read Macro Names.vi"("error in (no error)"=w493, "App Data Directory"=w488) -> ("error out"=w492:errorcluster, "Macro Names"=w489:string[])  [unwired: 8 in]
        n217 = Sort 1D Array(array=w489) -> (sorted array=w487:string[])
        n218 = Bundle By Name(cluster=w490, "Macro Names"=w487) -> (w491:T5)
        n219 = property on="Macro Name" class="CmbBox"("Strings[]"=w487) -> ()  [unwired: 2 in, 2 out]
      }
      frame "UI: Display Macro" {
        n220 = Unbundle By Name(w501) -> ("Macro.New"=w500:T6, "Macro.New.Config.Description"=w499:string, "Macro.New.Config.Activation Type"=w498:enum32{"Hotkey", "Automatic"}, "Macro.New.Config.N"=w497:i32)
        n221 = call "Display Data to Table.vi"("Macro"=w500) -> ("Metadata"=→"Metadata":string, "Macro Steps"=w494:string[][])  [unwired: 9 in]
        n222 = local write "Description"(w499) -> ()
        n223 = local write "Activation Type"(w498) -> ()
        n224 = local write "N"(w497) -> ()
        n225 = property on="Macro Steps" class="MCListbox (strict)"("ItemNames"=w494) -> ()  [unwired: 2 in, 2 out]
      }
      frame "UI: Update Status" {
        n226 = case shown="\"Abort Listen\"" w503 {
          tunnel: w504 -> [_ _ w514 w520 w526 w532 w538 _ _ _]
          tunnel: ["Idle" "Listening for hotkey press" w508 w515 w521 w527 w533 "Macro saved" ("Status") "Macro deleted" ("Status") "Macro restored to last save" ("Status")] -> w502
          frame "Idle", Default {
          }
          frame "Listen" {
          }
          frame "Step" {
            n227 = Unbundle By Name(w514) -> ("Macro.New"=w513:T6, "Step"=w512:i32, "n"=w511:i32, "Rcount"=w510:i32, "Start Time"=w509:timestamp)
            n228 = call "Build Status Message.vi"("Start Time"=w509, "Step Repeat"=w510, "Macro Repeat"=w511, "Step"=w512, "Macro"=w513) -> ("Status"=w508:string)  [unwired: 6 in]
          }
          frame "Complete Idle" {
            n229 = Unbundle By Name(w520) -> ("Start Time"=w518:timestamp)
            n230 = Get Date/Time In Seconds() -> (seconds since 1Jan1904=w517:timestamp)
            n231 = Subtract(x=w517, y=w518) -> (x-y=w516:dbl)
            n232 = Format Into String(format string="Macro completed in %.3t s.\nIdle", w516) -> (resulting string=w515:string)  [unwired: 2 in, 1 out]
          }
          frame "Complete Listen" {
            n233 = Unbundle By Name(w526) -> ("Start Time"=w524:timestamp)
            n234 = Get Date/Time In Seconds() -> (seconds since 1Jan1904=w523:timestamp)
            n235 = Subtract(x=w523, y=w524) -> (x-y=w522:dbl)
            n236 = Format Into String(format string="Macro completed in %.3t s.\nListening for hotkey press", w522) -> (resulting string=w521:string)  [unwired: 2 in, 1 out]
          }
          frame "Abort Idle" {
            n237 = Unbundle By Name(w532) -> ("Start Time"=w530:timestamp)
            n238 = Get Date/Time In Seconds() -> (seconds since 1Jan1904=w529:timestamp)
            n239 = Subtract(x=w529, y=w530) -> (x-y=w528:dbl)
            n240 = Format Into String(format string="Macro aborted after %.3t s.\nIdle", w528) -> (resulting string=w527:string)  [unwired: 2 in, 1 out]
          }
          frame "Abort Listen" {
            n241 = Unbundle By Name(w538) -> ("Start Time"=w536:timestamp)
            n242 = Get Date/Time In Seconds() -> (seconds since 1Jan1904=w535:timestamp)
            n243 = Subtract(x=w535, y=w536) -> (x-y=w534:dbl)
            n244 = Format Into String(format string="Macro aborted after %.3t s.\nListening for hotkey press", w534) -> (resulting string=w533:string)  [unwired: 2 in, 1 out]
          }
          frame "Save" {
          }
          frame "Delete" {
          }
          frame "Restore" {
          }
        }
        "Status" <- w502
      }
      frame "UI: Wait" {
        n245 = Unbundle By Name(w547) -> ("Keyboard"=w545:refnum<k1>, "Hotkey Values"=w544:T10)
        n246 = call "Check for Hotkey Press.vi"("Hotkey Type"=Hotkey_Type."Abort Hotkey", "error in (no error)"=w550, "Hotkeys"=w544, "Keyboard"=w545) -> ("error out"=w546:errorcluster, "Pressed?"=w542:bool)  [unwired: 5 in, 1 out]
        n247 = call "Timer FGV.vi"("Mode"=FGV_Actions."Read", "error in (no error)"=w546) -> ("error out"=w553:errorcluster, "Expired?"=w551:bool)  [unwired: 7 in, 1 out]
        n248 = case "Abort pressed?" shown="True" w542 {
          tunnel: w551 -> [w557 _]
          tunnel: [w554 "Macro: Process >> Abort" ("t")] -> w549
          frame False {
            n249 = Select(t="Macro: Process >> Step", s=w557, f="UI: Wait") -> (s? t:f=w554:string)
          }
          frame True {
          }
        }
        n250 = call "Enqueue Multiple States.vi"("queue in"=w548, "State(s) at Back"=w549) -> ()  [unwired: 13 in, 1 out]
      }
      frame "UI: Listen" {
        n251 = Unbundle By Name(w566) -> ("Keyboard"=w571:refnum<k1>, "Hotkey Values"=w561:T10)
        n252 = call "Stall Data Flow.vim"("value in"=w571, "milliseconds to wait"=u32 1) -> ("value out"=w569:refnum<k1>)  [unwired: 1 out]
        n253 = call "Check for Hotkey Press.vi"("Hotkey Type"=Hotkey_Type."Macro Hotkey", "error in (no error)"=w567, "Hotkeys"=w561, "Keyboard"=w569) -> ("error out"=w562:errorcluster, "Pressed?"=w559:bool)  [unwired: 5 in, 1 out]
        n254 = Select(t="Macro: Process >> Start", s=w559, f="UI: Listen" ("string")) -> (s? t:f=w565:string)
        n255 = call "Enqueue Multiple States.vi"("queue in"=w563, "State(s) at Back"=w565) -> ()  [unwired: 13 in, 1 out]
      }
      frame "UI: Settings" {
        n256 = call "Change Settings.vi"("error in (no error)"=w573) -> ("error out"=w572:errorcluster)  [unwired: 10 in]
      }
      frame "UI: Prompt for Save" {
        n257 = Unbundle By Name(w585) -> ("Macro Names"=w577:string[], "Macro.Name"=w576:string)
        n258 = Search 1D Array(1D array=w577, element=w576) -> (index of element=w575:i32)  [unwired: 1 in]
        n259 = Greater Or Equal To 0?(x=w575) -> (x >= 0?=w581:bool)
        n260 = call "Overwrite?"("Enable"=w581) -> ("Overwrite"=w580:bool)  [unwired: 9 in, 1 out]
        n261 = Implies(1:w580, 2:w581) -> (0:w579:bool)
        n262 = Select(t="Data: Bundle Macro\nData: Save Macro\nUI: Populate Macros\nUI: Update Status >> Save\nUI: Interlocks", s=w579, f="") -> (s? t:f=w582:string)
        n263 = call "Enqueue Multiple States.vi"("queue in"=w586, "State(s) at Back"=w582) -> ()  [unwired: 13 in, 1 out]
      }
      frame "UI: Confirm Exit" {
        n264 = Unbundle By Name(w595) -> ("Macro.New"=w591:T6, "Macro.Saved"=w592:T6)
        n265 = Not Equal?(x=w591, y=w592) -> (x != y?=w590:bool)
        n266 = call "Exit anyway?"("Enable"=w590) -> ("Exit"=w594:bool)  [unwired: 9 in, 1 out]
        n267 = Implies(1:w594, 2:w590) -> (0:w588:bool)
        n268 = case shown="True" w588 {
          tunnel: w593 -> [w596 w600]
          tunnel: [w596 w599] -> w589
          tunnel: w587 -> [_ w598]
          frame False {
          }
          frame True {
            n269 = Generate User Event(user event=w598, event data cluster=TRUE ("event data"), error in=w600) -> (error out=w599:errorcluster)  [unwired: 1 in, 1 out]
          }
        }
      }
      frame "---------- Macro ----------" {
        # "Do not put any code in this frame.\n(It is a separator no-op. You can make a copy of this frame to create a new Macro frame)"
      }
      frame "Macro: Initialize" {
        w603 = "Data: Initialize\nData: Bundle Refs\nInitialize Core Data\nUI: Initialize\nData: Get Hotkey\nUI: Populate Macros\nUI: Interlocks\nUI: Front Panel State >> Open\nData: Migrate Config\nUI: Update Status >> Idle"  # Data: Initialize Data: Bundle Refs Initialize Core Data UI: Initialize Data: Get Hotkey UI: Populate Macros UI: Interlocks UI: Front Panel State >> Open Data: Migrate Config UI: Update Status >> Idle
        # "Initialization Macro\n(This is called once, when the VI starts)"
        n270 = call "Enqueue Multiple States.vi"("State(s) at Front"=w603, "queue in"=w606) -> ()  [unwired: 13 in, 1 out]
      }
      frame "Macro: Process" {
        n271 = case shown="\"Start\", Default" w611 {
          tunnel: w608 -> [w619 w626 w632 w647 w651 w657]
          tunnel: [w622 w625 w630 w645 w651 w657] -> w610
          tunnel: [w613 "UI: Update Status >> Step\nProcess: Perform Step" w628 w643 w652 w658] -> w609
          frame "Start", Default {
            w621 = 0 ("Step")
            n272 = Unbundle By Name(w619) -> ("Macro.New.Config.Activation Type"=w614:enum32{"Hotkey", "Automatic"})
            n273 = Equal?(x=w614, y=enum32{"Hotkey", "Automatic"}."Hotkey") -> (x = y?=w618:bool)
            n274 = Get Date/Time In Seconds() -> (seconds since 1Jan1904=w620:timestamp)
            n275 = Select(t="UI: Interlocks\nUI: Update Status >> Listen\nUI: Listen", s=w618, f="UI: Interlocks\nUI: Update Status >> Step\nProcess: Perform Step") -> (s? t:f=w613:string)
            n276 = Bundle By Name(cluster=w619, "Step"=w621, "n"=w621, "Rcount"=w621, "Start Time"=w620) -> (w622:T5)
          }
          frame "Repeat" {
            w623 = 0 ("Step")
            n277 = Bundle By Name(cluster=w626, "Step"=w623, "Rcount"=w623) -> (w625:T5)
          }
          frame "Step" {
            n278 = Unbundle By Name(w632) -> ("Step"=w637:i32, "Macro.New.Steps"=w635:T8[])
            n279 = Array Size(array=w635) -> (size(s)=w636:i32)
            n280 = Increment(x=w637) -> (x+1=w631:i32)
            n281 = Greater Or Equal?(x=w631, y=w636) -> (x >= y?=w634:bool)
            n282 = Select(t="Macro: Process >> Complete", s=w634, f="UI: Update Status >> Step\nProcess: Perform Step") -> (s? t:f=w628:string)
            n283 = Bundle By Name(cluster=w632, "Step"=w631, "Rcount"=0) -> (w630:T5)
          }
          frame "Complete" {
            n284 = Unbundle By Name(w647) -> ("n"=w649:i32, "Macro.New.Config.N"=w638:i32)
            n285 = Increment(x=w649) -> (x+1=w646:i32)
            n286 = Greater?(x=w646, y=w638) -> (0:w641:bool)
            n287 = Not Equal?(x=w638, y=-1) -> (x != y?=w640:bool)
            n288 = And(x=w641, y=w640) -> (x .and. y?=w639:bool)
            n289 = Select(t="Macro: Process >> End", s=w639, f="Macro: Process >> Repeat") -> (s? t:f=w643:string)
            n290 = Bundle By Name(cluster=w647, "n"=w646) -> (w645:T5)
          }
          frame "End" {
            n291 = Unbundle By Name(w651) -> ("Macro.New.Config.Activation Type"=w650:enum32{"Hotkey", "Automatic"})
            n292 = case shown="\"Automatic\"" w650 {
              tunnel: ["UI: Update Status >> Complete Listen\nUI: Listen" "UI: Update Status >> Complete Idle"] -> w652
              frame "Hotkey" {
              }
              frame "Automatic" {
                n293 = property on="Start/Stop" class="Bool (strict)"("Val(Sgnl)"=FALSE ("Value (Signaling)")) -> ()  [unwired: 2 in, 2 out]
              }
            }
          }
          frame "Abort" {
            n294 = Unbundle By Name(w657) -> ("Macro.New.Config.Activation Type"=w656:enum32{"Hotkey", "Automatic"})
            n295 = case shown="\"Automatic\"" w656 {
              tunnel: ["UI: Update Status >> Abort Listen\nUI: Listen" "UI: Update Status >> Abort Idle"] -> w658
              frame "Hotkey" {
              }
              frame "Automatic" {
                n296 = property on="Start/Stop" class="Bool (strict)"("Val(Sgnl)"=FALSE ("Value (Signaling)")) -> ()  [unwired: 2 in, 2 out]
              }
            }
          }
        }
        n297 = call "Enqueue Multiple States.vi"("queue in"=w607, "State(s) at Back"=w609) -> ()  [unwired: 13 in, 1 out]
      }
      frame "Macro: Exit" {
        # "Exit Macro\n(This is called once, when the VI exits)"
        n298 = Unbundle By Name(w670) -> ("Core.Close Panel on Exit?"=w669:bool)
        n299 = property on="Macro Steps" class="MCListbox (strict)"("TopLeft"=T13 {"Row"=0, "Column"=0} ("Index Values")) -> ()  [unwired: 2 in, 2 out]
        n300 = property on="Macro Steps" class="MCListbox (strict)"("ItemNames"=string[][] [] ("Item Names")) -> ()  [unwired: 2 in, 2 out]
        n301 = Select(t="UI: Front Panel State >> Close", s=w669, f="") -> (s? t:f=w664:string)
        n302 = call "Enqueue Multiple States.vi"("State(s) at Front"=w664, "queue in"=w665, "State(s) at Back"="Data: Cleanup\nExit") -> ()  [unwired: 12 in, 1 out]
      }
      frame "---------- Process ----------" {
      }
      frame "Process: Perform Step" {
        n303 = in-place {
          in-place-border: [w686] -> w674
          n304 = in-place-cluster #3(w676) -> ("Rcount"=w687:i32)
          n305 = Increment(x=w687) -> (x+1=w686:i32)
          n306 = in-place-cluster #3("Rcount"=w686) -> (w675:T5)
        }
        n307 = Unbundle By Name(w676) -> ("Macro.New.Steps"=w685:T8[], "Step"=w684:i32, "Hotkey Values"=w679:T10, "Keyboard"=w680:refnum<k1>)
        n308 = Index Array(array=w685, index=w684) -> (element=w678:T8)
        n309 = call "Perform Step.vi"("Repeat Count"=w674, "error in (no error)"=w682, "Keyboard"=w680, "Hotkeys"=w679, "Step"=w678) -> ("error out"=w681:errorcluster, "State(s)"=w677:string)  [unwired: 5 in]
        n310 = call "Enqueue Multiple States.vi"("queue in"=w683, "State(s) at Back"=w677) -> ()  [unwired: 13 in, 1 out]
      }
    }
  }
  n311 = Merge Errors(w9, w8) -> (w10:errorcluster)
  n312 = Release Queue(queue=w11, error in (no error)=w10) -> (error out=→"error out":errorcluster)  [unwired: 1 in, 2 out]
